vi "NISE.Commit Properties (Generic).vi"(0 "SLSC Interface in":refnum<class "SLSC Interface.lvclass">, 5 "resources":string, 11 "error in (no error)":errorcluster) -> (4 "SLSC Interface out":refnum<class "SLSC Interface.lvclass">, 15 "error out":errorcluster)   [LabVIEW 2016, in "SLSC Interface.lvclass"]
uses:
  SLSC Interface.lvclass
  SLSC Interface.lvclass/SLSC Interface.ctl
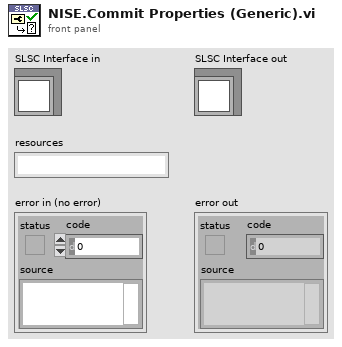
[diagram p1: front panel]
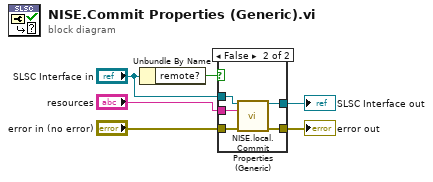
[diagram p0: block diagram]
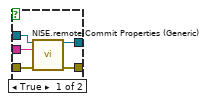
[diagram p2: hidden frame]
diagram:
  n1 = Unbundle By Name("SLSC Interface in") -> ("remote?"=w6:bool)
  n2 = case shown="False" w6 {
    tunnel: "SLSC Interface in" -> [w11 w16]
    tunnel: [w10 w15] -> w5
    tunnel: "resources" -> [w9 w14]
    tunnel: "error in (no error)" -> [w8 w13]
    tunnel: [w7 w12] -> w2
    frame True {
      n3 = call "NISE.remote.Commit Properties (Generic).vi"("SLSC Remote in"=w11, "resources"=w9, "error in (no error)"=w8) -> ("SLSC Remote out"=w10:refnum<class "SLSC Interface.lvclass">, "error out"=w7:errorcluster)  [unwired: 11 in]
    }
    frame False {
      n4 = call "NISE.local.Commit Properties (Generic).vi"("SLSC Local in"=w16, "resources"=w14, "error in (no error)"=w13) -> ("SLSC Local out"=w15:refnum<class "SLSC Interface.lvclass">, "error out"=w12:errorcluster)  [unwired: 11 in]
    }
  }
  "error out" <- w2
  "SLSC Interface out" <- w5
